vi "sequentialDataWriter.vi"() -> ()   [LabVIEW 2012]
uses:
  ActiveMQBroker/ActiveMQBroker.lvclass
panel:
  in  "stopWriter":bool
  in  "topic":string="testTopic"
  in  "port":string="61616"
  in  "host":string="localhost"
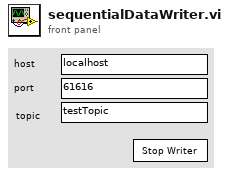
[diagram p1: front panel]
types:
  T1 = enum32{"invalid app kind", "Development System", "Run Time System", "Student Edition", "Embedded LabVIEW", "Evaluation", "Custom"}
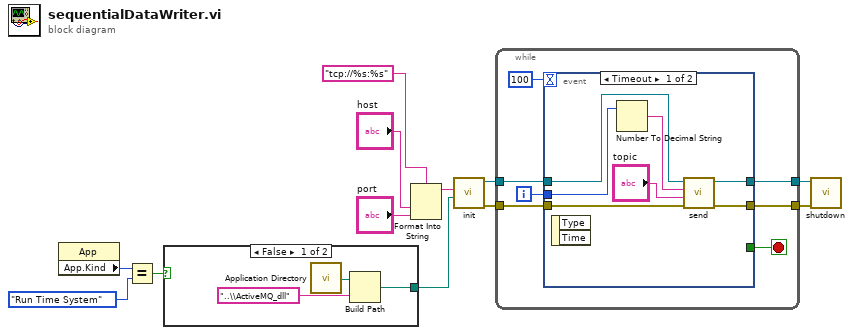
[diagram p0: block diagram]
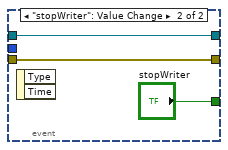
[diagram p2: hidden frame]
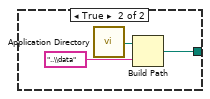
[diagram p3: hidden frame]
diagram:
  n1 = property class="App"() -> ("App.Kind"=w9:T1)  [unwired: 2 in, 2 out]
  n2 = Equal?(x=w9, y=T1."Run Time System") -> (x = y?=w7:bool)
  n3 = case shown="False" w7 {
    tunnel: [w13 w16] -> w12
    frame False {
      n4 = call <vilib>:"Application Directory.vi"() -> ("Application Directory"=w14:path)
      n5 = Build Path(base path=w14, name or relative path="..\\ActiveMQ_dll") -> (appended path=w13:path)
    }
    frame True {
      n6 = call <vilib>:"Application Directory.vi"() -> ("Application Directory"=w18:path)
      n7 = Build Path(base path=w18, name or relative path="..\\data") -> (appended path=w16:path)
    }
  }
  n8 = Format Into String(format string="tcp://%s:%s", "host", "port") -> (resulting string=w5:string)  [unwired: 2 in, 1 out]
  n9 = call "init.vi"("activeMQ_dll_directory"=w12, "brokerConnectionString"=w5) -> ("error out"=w1:errorcluster, "ActiveMQBroker out"=w2:refnum<class "ActiveMQBroker.lvclass">)  [unwired: 7 in, 1 out]
  n10 = while {
    tunnel: [w25] -> w11
    tunnel: [w24] -> w10
    tunnel: w2 -> [w23]
    tunnel: w1 -> [w22]
    i -> [w19]
    stop <- w21 stop-if-true
    n11 = event shown="[0] Timeout" {
      selector: _ -> [_ _]
      dyn-events: _ -> [_ _]
      timeout: 100 -> [_ _]
      tunnel: [w32 w34] -> w25
      tunnel: [w31 w33] -> w24
      tunnel: w23 -> [w29 w34]
      tunnel: w22 -> [w28 w33]
      tunnel: [_ "stopWriter"] -> w21
      tunnel: w19 -> [w27 _]
      event Timeout {
        n12 = event-data() -> ()  [unwired: 1 in, 2 out]
        n13 = Number To Decimal String(number=w27) -> (decimal integer string=w26:string)  [unwired: 1 in]
        n14 = call-dynamic "send.vi"("error in (no error)"=w28, "topic"="topic", "message"=w26, "ActiveMQBroker in"=w29) -> ("error out"=w31:errorcluster, "ActiveMQBroker out"=w32:refnum<class "ActiveMQBroker.lvclass">)  [unwired: 6 in]
      }
      event "stopWriter": Value Change {
        n15 = event-data() -> ()  [unwired: 1 in, 2 out]
      }
    }
  }
  n16 = call-dynamic "shutdown.vi"("error in (no error)"=w10, "ActiveMQBroker in"=w11) -> ()  [unwired: 8 in, 2 out]
